vi "DSF.Engine.Status.Framework.Performance.Get Rx Start Time.vi"(11 "Framework Performance in":refnum<class "DSF.Engine.Status.Framework.Performance.lvclass">) -> (2 "Rx start time":u32 format="%d us", 3 "Framework Performance out":refnum<class "DSF.Engine.Status.Framework.Performance.lvclass">)   [LabVIEW 2017, in "DSF.Engine.lvlib" / "DSF.Engine.Status.Framework.Performance.lvclass"]
uses:
  DSF.Engine.Status.Framework.Performance.lvclass
  DSF.Engine.Status.Framework.Performance.lvclass/DSF.Engine.Status.Framework.Performance.ctl
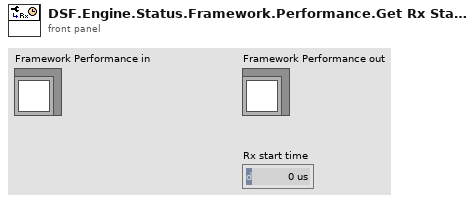
[diagram p1: front panel]
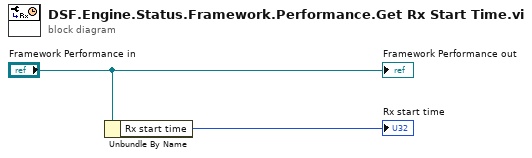
[diagram p0: block diagram]
diagram:
  n1 = Unbundle By Name("Framework Performance in") -> ("Rx start time"=→"Rx start time":u32)
  "Framework Performance out" <- "Framework Performance in"
